vi "GetAllValues.vi"(0 "object in":refnum<class "Node.lvclass">, 5 "Error In":errorcluster) -> (14 "object out":refnum<class "Node.lvclass">, 16 "Values":string, 19 "Error Out":errorcluster)   [LabVIEW 2024, in "Node.lvclass"]
uses:
  Node.lvclass
  Node.lvclass/Node.ctl
  Element_interface/Element.lvclass
panel:
  # "Connector Pane"
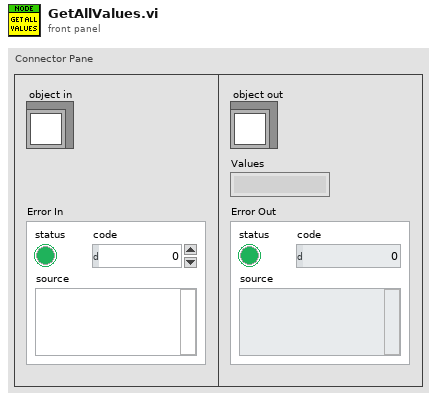
[diagram p1: front panel]
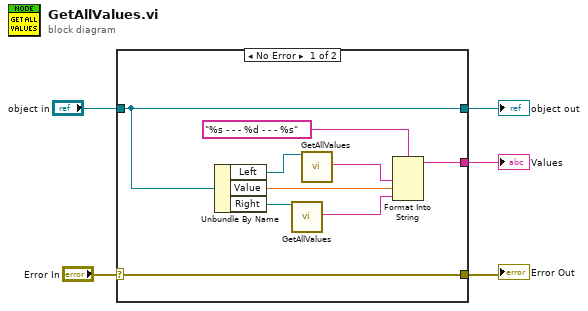
[diagram p0: block diagram]
diagram:
  n1 = case shown="No Error" "Error In" {
    selector: "Error In" -> [w14 w16]
    tunnel: [w14 w16] -> w4
    tunnel: [w8 w15] -> w2
    tunnel: "object in" -> [w8 w15]
    tunnel: [w9 _] -> w1
    frame No Error {
      n2 = Unbundle By Name(w8) -> ("Left"=w12:refnum<class "Element.lvclass">, "Value"=w6:dbl, "Right"=w11:refnum<class "Element.lvclass">)
      n3 = call-dynamic "GetAllValues.vi"("object in"=w11) -> ("Values"=w10:string)  [unwired: 16 in, 2 out]
      n4 = call-dynamic "GetAllValues.vi"("object in"=w12) -> ("Values"=w7:string)  [unwired: 16 in, 2 out]
      n5 = Format Into String(format string="%s - - - %d - - - %s", w7, w6, w10) -> (resulting string=w9:string)  [unwired: 2 in, 1 out]
    }
    frame Error {
    }
  }
  "Error Out" <- w4
  "object out" <- w2
  "Values" <- w1
